vi "Read VI Path.vi"(8 "error in (no error)":errorcluster, 11 "VIConverter in":refnum<class "VIConverter.lvclass">) -> (0 "error out":errorcluster, 2 "VI Path":path, 3 "VIConverter out":refnum<class "VIConverter.lvclass">)   [LabVIEW 2017, in "VIConverter.lvclass"]
uses:
  VIConverter.lvclass
  VIConverter.lvclass/VIConverter.ctl
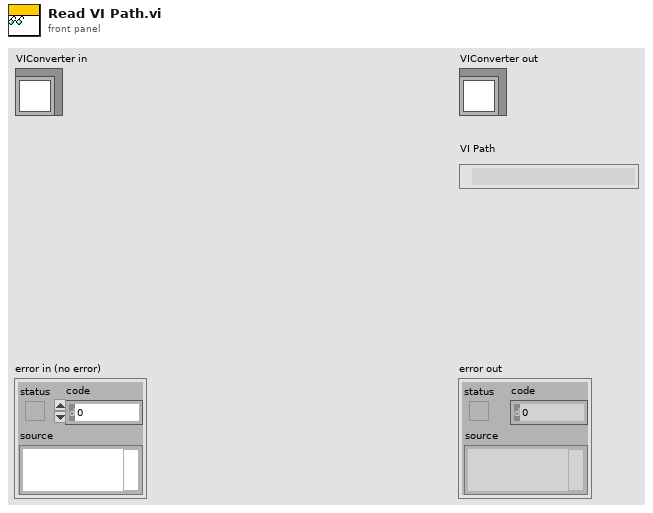
[diagram p1: front panel]
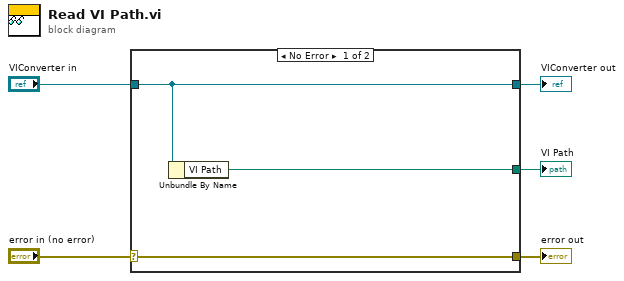
[diagram p0: block diagram]
diagram:
  n1 = case shown="No Error" "error in (no error)" {
    selector: "error in (no error)" -> [w8 w9]
    tunnel: [w8 w9] -> w4
    tunnel: [w7 w10] -> w2
    tunnel: "VIConverter in" -> [w7 w10]
    tunnel: [w6 _] -> w1
    frame No Error {
      n2 = Unbundle By Name(w7) -> ("VI Path"=w6:path)
    }
    frame Error {
    }
  }
  "error out" <- w4
  "VIConverter out" <- w2
  "VI Path" <- w1
